vi "2D Path to Points.vi"(8 "Number Of Points":i32=100, 9 "Forward":bool, 10 "Spline Y":dbl[](array[numeric]), 11 "Spline X":dbl[](array[numeric])) -> (3 "Points":T1(array[cluster]))   [LabVIEW 2016]
uses:
  <vilib>/Analysis/polynomials.llb/nth Derivative of Polynomial (DBL).vi
  <vilib>/Analysis/polynomials.llb/Scalar Polynomial Evaluation (DBL).vi
  <vilib>/Analysis/NI_AALPro.lvlib
panel:
  # "s is not seconds! it is a special time unit"
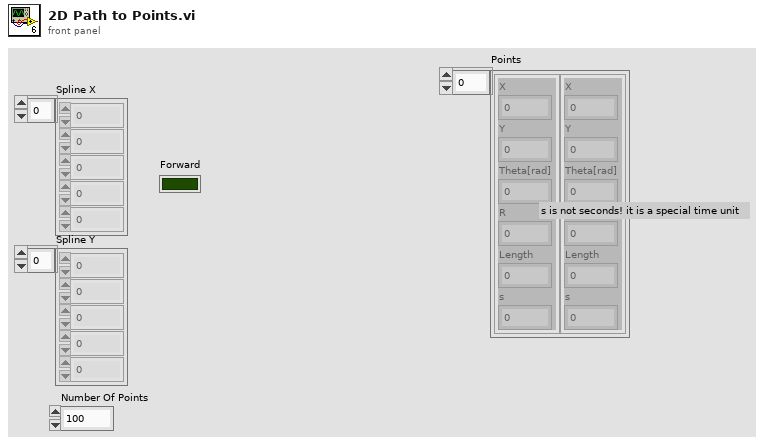
[diagram p1: front panel]
types:
  T1 = cluster{"X":dbl, "Y":dbl, "Theta[rad]":dbl, "R":dbl, "Length":dbl, "s":dbl}[]
  T2 = cluster{"X":dbl, "Y":dbl, "Theta[rad]":dbl, "R":dbl, "Length":dbl, "s":dbl}
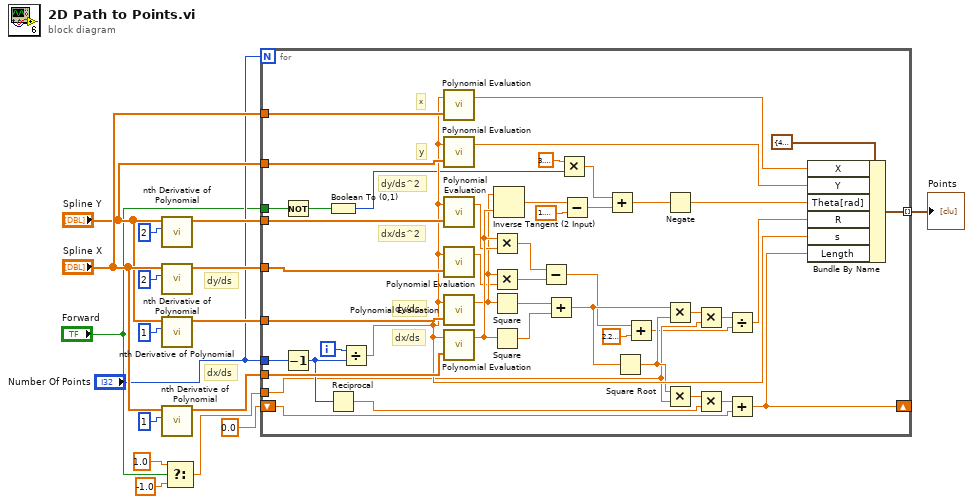
[diagram p0: block diagram]
diagram:
  # "dy/ds"
  # "dx/ds"
  n1 = call-poly <vilib>:"nth Derivative of Polynomial.vi"("order"=2, "P(x)"="Spline Y") -> ("Nth Derivative of P(x)"=w9:dbl[])  [unwired: 8 in, 1 out]
  n2 = call-poly <vilib>:"nth Derivative of Polynomial.vi"("order"=2, "P(x)"="Spline X") -> ("Nth Derivative of P(x)"=w8:dbl[])  [unwired: 8 in, 1 out]
  n3 = call-poly <vilib>:"nth Derivative of Polynomial.vi"("order"=1, "P(x)"="Spline Y") -> ("Nth Derivative of P(x)"=w14:dbl[])  [unwired: 8 in, 1 out]
  n4 = call-poly <vilib>:"nth Derivative of Polynomial.vi"("order"=1, "P(x)"="Spline X") -> ("Nth Derivative of P(x)"=w15:dbl[])  [unwired: 8 in, 1 out]
  n5 = Select(t=1.0, s="Forward", f=-1.0) -> (s? t:f=w5:dbl)
  n6 = for {
    N: "Number Of Points" -> [_]
    tunnel: "Spline X" -> [w63]
    tunnel: "Spline Y" -> [w62]
    tunnel: w15 -> [w57]
    tunnel: w14 -> [w56]
    tunnel: [w58] -> w4 mode=indexing
    tunnel: w9 -> [w45]
    tunnel: w8 -> [w46]
    tunnel: w5 -> [w30]
    shift-right: [w32] -> _
    shift-left: 0.0 -> [w33]
    tunnel: "Number Of Points" -> [w38]
    tunnel: "Forward" -> [w25]
    i -> [w61]
    # "dx/ds^2"
    # "dy/ds^2"
    # "dy/ds"
    # "dx/ds"
    # "y"
    # "x"
    n7 = Not(x=w25) -> (.not. x?=w24:bool)
    n8 = Decrement(x=w38) -> (x-1=w36:i32)
    n9 = Boolean To (0,1)(Boolean=w24) -> (0, 1=w23:i16)
    n10 = Reciprocal(x=w36) -> (1/x=w35:dbl)
    n11 = Divide(x=w61, y=w36) -> (x/y=w44:dbl)
    n12 = call-poly <vilib>:"Polynomial Evaluation.vi"("P(x)"=w63, "a"=w44) -> ("P(a)"=w60:dbl)  [unwired: 1 out]
    n13 = call-poly <vilib>:"Polynomial Evaluation.vi"("P(x)"=w62, "a"=w44) -> ("P(a)"=w59:dbl)  [unwired: 1 out]
    n14 = call-poly <vilib>:"Polynomial Evaluation.vi"("P(x)"=w45, "a"=w44) -> ("P(a)"=w49:dbl)  [unwired: 1 out]
    n15 = call-poly <vilib>:"Polynomial Evaluation.vi"("P(x)"=w46, "a"=w44) -> ("P(a)"=w47:dbl)  [unwired: 1 out]
    n16 = call-poly <vilib>:"Polynomial Evaluation.vi"("P(x)"=w56, "a"=w44) -> ("P(a)"=w48:dbl)  [unwired: 1 out]
    n17 = call-poly <vilib>:"Polynomial Evaluation.vi"("P(x)"=w57, "a"=w44) -> ("P(a)"=w50:dbl)  [unwired: 1 out]
    n18 = Multiply(x=w50, y=w49) -> (x*y=w43:dbl)
    n19 = Multiply(x=w48, y=w47) -> (x*y=w42:dbl)
    n20 = Square(x=w48) -> (x^2=w54:dbl)
    n21 = Square(x=w50) -> (x^2=w55:dbl)
    n22 = Inverse Tangent (2 Input)(1:w50, 2:w48) -> (0:w41:dbl)
    n23 = Subtract(x=w43, y=w42) -> (x-y=w20:dbl)
    n24 = Add(x=w54, y=w55) -> (x+y=w53:dbl)
    n25 = Multiply(x=3.141592653589793, y=w23) -> (x*y=w21:dbl)
    n26 = Subtract(x=w41, y=1.5707963267948966) -> (x-y=w29:dbl)
    n27 = Add(x=w21, y=w29) -> (x+y=w26:dbl)
    n28 = Square Root(x=w53) -> (sqrt(x)=w37:dbl)
    n29 = Add(x=w20, y=2.220446049250313e-16) -> (x+y=w18:dbl)
    n30 = Negate(x=w26) -> (-x=w27:dbl)
    n31 = Multiply(x=w53, y=w37) -> (x*y=w52:dbl)
    n32 = Multiply(x=w37, y=w30) -> (x*y=w31:dbl)
    n33 = Multiply(x=w52, y=w30) -> (x*y=w51:dbl)
    n34 = Multiply(x=w31, y=w35) -> (x*y=w34:dbl)
    n35 = Divide(x=w51, y=w18) -> (x/y=w40:dbl)
    n36 = Add(x=w34, y=w33) -> (x+y=w32:dbl)
    n37 = Bundle By Name(cluster=T2 {"X"=40.0149, "Y"=49.78427277290001, "Theta[rad]"=1.7171484123050091, "R"=-1.3413244230140104, "Length"=0.0, "s"=0.99} ("Points 2"), "X"=w60, "Y"=w59, "Theta[rad]"=w27, "R"=w40, "s"=w44, "Length"=w32) -> (w58:T2)
  }
  "Points" <- w4
